vi "Send Configure AC Line Trigger Slope [AT].vi"(7 "Message Priority (Normal)":T1=enum."Normal", 8 "error in (no error)":errorcluster, 10 "ac line trigger slope (Positive)":i32(ring)=1 items=["Positive"=1, "Negative"=2, "Either"=3], 11 "Message Enqueuer":refnum<class "Message Enqueuer.lvclass">) -> (0 "error out":errorcluster, 3 "Message Enqueuer out":refnum<class "Message Enqueuer.lvclass">)   [LabVIEW 2016, in "CS++Scope.lvlib" / "Configure AC Line Trigger Slope [AT] Msg.lvclass"]
doc: "Sends the <B>CS++Scope.lvlib:Configure AC Line Trigger Slope [AT] Msg.lvclass</B> message.\n\n<B>CS++Scope.lvlib:CS++Scope.lvclass:Configure AC Line Trigger Slope [AT].vi</B> Description:\n\nThis VI configures the slope of the AC Line trigger.\n\nNote (1) This VI affects instrument behavior only if the trigger type is IVISCOPE_VAL_AC_LINE_TRIGGER. Call the IviScope Configure Trigger VI to set the trigger type before calling this VI.\n(2) This VI is part of the IviScopeAcLineTrigger [AT] extension group."
uses:
  Configure AC Line Trigger Slope [AT] Msg.lvclass
  <vilib>/ActorFramework/Message Enqueuer/Message Enqueuer.lvclass
  <vilib>/ActorFramework/Message Enqueuer/Message Priority.ctl
  C:/Program Files (x86)/National Instruments/LabVIEW 2016/vi.lib/ActorFramework/Message/Message.lvclass
  Configure AC Line Trigger Slope [AT] Msg.lvclass/Configure AC Line Trigger Slope [AT] Msg.ctl
  <vilib>/ActorFramework/Message Enqueuer/Message Enqueuer.lvclass/Message Enqueuer.ctl
  <vilib>/ActorFramework/Message Priority Queue/Priority Enqueue.vi
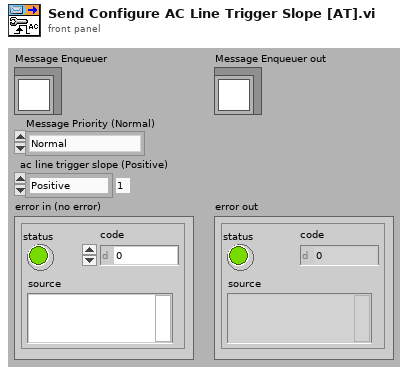
[diagram p1: front panel]
types:
  T1 = typedef "Actor Framework.lvlib/Message Enqueuer.lvclass/Message Priority.ctl" = enum16{"Low", "Normal", "High"}
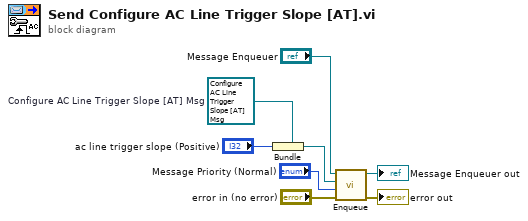
[diagram p0: block diagram]
diagram:
  w2 = refnum<class "Configure AC Line Trigger Slope [AT] Msg.lvclass"> refnum  # Configure AC Line Trigger Slope [AT] Msg
  n1 = Bundle(cluster=w2, "ac line trigger slope (Positive)") -> (w5:refnum<class "Configure AC Line Trigger Slope [AT] Msg.lvclass">)
  n2 = call <vilib>:"Enqueue.vi"("error in (no error)"="error in (no error)", "Message Priority (Normal)"="Message Priority (Normal)", "Message"=w5, "Message Enqueuer in"="Message Enqueuer") -> ("error out"=→"error out":errorcluster, "Message Enqueuer out"=→"Message Enqueuer out":refnum<class "Message Enqueuer.lvclass">)  [unwired: 6 in]
